vi "TimeFacade.vi"(0 "Data In":T4, 2 "Display State In":T2, 3 "Container State":T3) -> (6 "Data Out":T4, 7 "Display State Out":T2, 8 "Action":T1)   [LabVIEW 2018, in "Ui.lvlib" / "Time.xctl"]
uses:
  Time.xctl
  TimeData.ctl
  <vilib>/_xctls/Container State.ctl
  TimeState.ctl
  <vilib>/_xctls/Action.ctl
  <vilib>/_xctls/XControlSupport.lvlib
panel:
  in  "Knob":dbl(knob) min=0.0001 max=10000.0 step=0.001 scale=10.0..10000.0
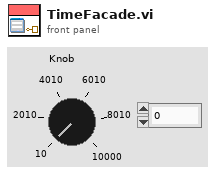
[diagram p1: front panel]
types:
  T1 = typedef "XControlSupport.lvlib/Action.ctl" = cluster{"Data Changed?":bool, "State Changed?":bool, "Action Name":string}
  T2 = typedef "Ui.lvlib/Time.xctl/TimeState.ctl" = cluster{"Enum":enum16{"Time", "Frequency"}}
  T3 = typedef "XControlSupport.lvlib/Container State.ctl" = cluster{"Indicator?":bool, "Run Mode?":bool, " Refnum":refnum<vi>}
  T4 = typedef "Ui.lvlib/Time.xctl/TimeData.ctl" = i64
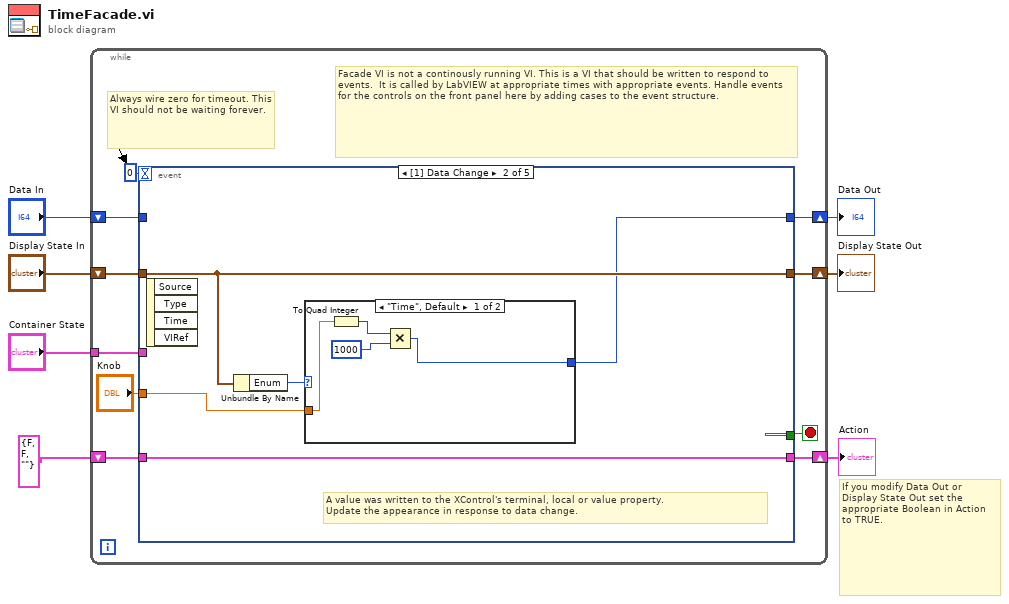
[diagram p0: block diagram]
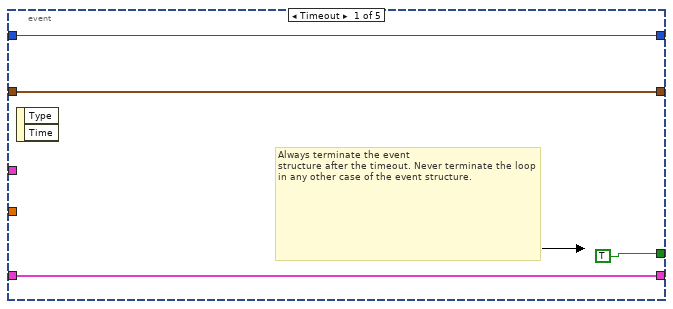
[diagram p2: hidden frame]
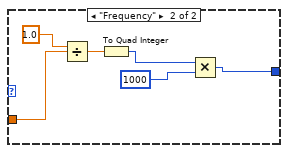
[diagram p3: hidden frame]
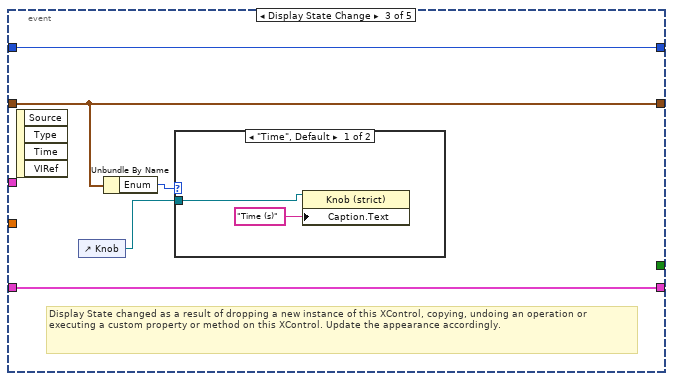
[diagram p4: hidden frame]
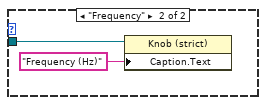
[diagram p5: hidden frame]
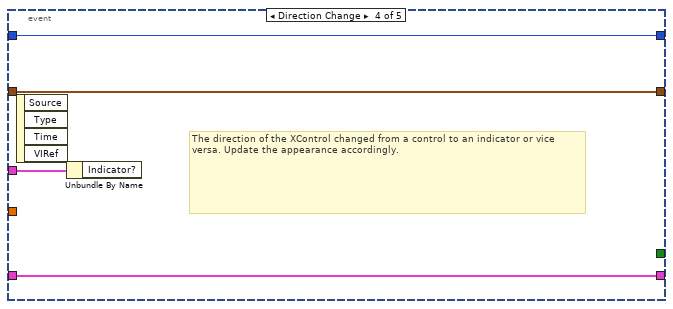
[diagram p6: hidden frame]
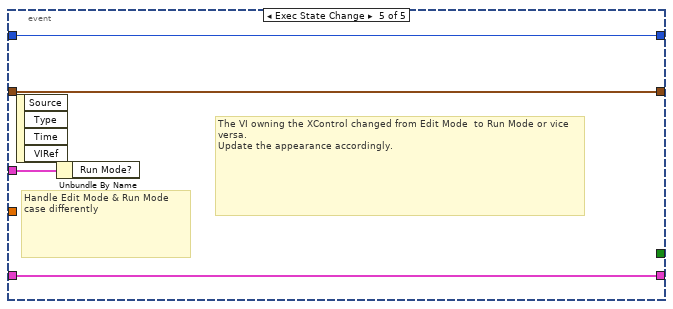
[diagram p7: hidden frame]
diagram:
  # "If you modify Data Out or\nDisplay State Out set the\nappropriate Boolean in Action\nto TRUE."
  n1 = while {
    shift-right: [w16] -> w4
    shift-left: "Display State In" -> [w17]
    tunnel: "Container State" -> [w13]
    shift-right: [w11] -> w7
    shift-left: "Data In" -> [w12]
    shift-right: [w9] -> w2
    shift-left: T1 {"Data Changed?"=FALSE, "State Changed?"=FALSE, "Action Name"=""} ("Action") -> [w10]
    stop <- w15 stop-if-true
    # "Facade VI is not a continously running VI. This is a VI that should be written to respond to events.  It is called by LabVIEW at appropriate times with appropriate events. Handle events for the controls on the front panel here by adding cases to the event structure."
    # "Always wire zero for timeout. This\nVI should not be waiting forever."
    n2 = event shown="[1] Data Change" {
      selector: _ -> [_ _ _ _ _]
      dyn-events: _ -> [_ _ _ _ _]
      timeout: 0 -> [_ _ _ _ _]
      tunnel: w17 -> [w19 w26 w38 w48 w52]
      tunnel: [w19 w26 w38 w48 w52] -> w16
      tunnel: [TRUE _ _ _ _] -> w15
      tunnel: w13 -> [_ _ _ w49 w53]
      tunnel: w12 -> [w18 _ w41 w47 w51]
      tunnel: [w18 w24 w41 w47 w51] -> w11
      tunnel: [w20 w22 w40 w46 w50] -> w9
      tunnel: w10 -> [w20 w22 w40 w46 w50]
      tunnel: "Knob" -> [_ w23 _ _ _]
      event Timeout {
        # "Always terminate the event\nstructure after the timeout. Never terminate the loop in any other case of the event structure."
        n3 = event-data() -> ()  [unwired: 1 in, 2 out]
      }
      event Data Change {
        # "A value was written to the XControl's terminal, local or value property.\nUpdate the appearance in response to data change."
        n4 = event-data() -> ()  [unwired: 1 in, 4 out]
        n5 = Unbundle By Name(w26) -> ("Enum"=w25:enum16{"Time", "Frequency"})
        n6 = case shown="\"Time\", Default" w25 {
          tunnel: [w28 w32] -> w24
          tunnel: w23 -> [w27 w31]
          frame "Time", Default {
            n7 = To Quad Integer(1:w27) -> (0:w30:i64)
            n8 = Multiply(x=w30, y=i64 1000) -> (x*y=w28:i64)
          }
          frame "Frequency" {
            n9 = Divide(x=1.0, y=w31) -> (x/y=w35:dbl)
            n10 = To Quad Integer(1:w35) -> (0:w34:i64)
            n11 = Multiply(x=w34, y=i64 1000) -> (x*y=w32:i64)
          }
        }
      }
      event Display State Change {
        # "Display State changed as a result of dropping a new instance of this XControl, copying, undoing an operation or executing a custom property or method on this XControl. Update the appearance accordingly."
        n12 = event-data() -> ()  [unwired: 1 in, 4 out]
        n13 = control-ref of="Knob"() -> (w37:refnum<vi>)
        n14 = Unbundle By Name(w38) -> ("Enum"=w39:enum16{"Time", "Frequency"})
        n15 = case shown="\"Time\", Default" w39 {
          tunnel: w37 -> [w42 w44]
          frame "Time", Default {
            n16 = property on="Property Node" class="Knob (strict)"(reference=w42, "Caption.Text"="Time (s)") -> ()  [unwired: 1 in, 2 out]
          }
          frame "Frequency" {
            n17 = property on="Property Node" class="Knob (strict)"(reference=w44, "Caption.Text"="Frequency (Hz)") -> ()  [unwired: 1 in, 2 out]
          }
        }
      }
      event Direction Change {
        # "The direction of the XControl changed from a control to an indicator or vice versa. Update the appearance accordingly."
        n18 = event-data() -> ()  [unwired: 1 in, 4 out]
        n19 = Unbundle By Name(w49) -> ()  [unwired: 1 out]
      }
      event Exec State Change {
        # "The VI owning the XControl changed from Edit Mode  to Run Mode or vice versa.\nUpdate the appearance accordingly."
        # "Handle Edit Mode & Run Mode\ncase differently"
        n20 = event-data() -> ()  [unwired: 1 in, 4 out]
        n21 = Unbundle By Name(w53) -> ()  [unwired: 1 out]
      }
    }
  }
  "Display State Out" <- w4
  "Data Out" <- w7
  "Action" <- w2
